vi "SetEmbeddedName.vi"(8 "error in (no error)":errorcluster, 10 "Name":string, 11 "EmbeddedSMO in":refnum<class "EmbeddedSMO.lvclass">) -> (0 "error out":errorcluster, 3 "EmbeddedSMO out":refnum<class "EmbeddedSMO.lvclass">)   [LabVIEW 2016, in "EmbeddedSMO.lvclass"]
uses:
  EmbeddedSMO.lvclass
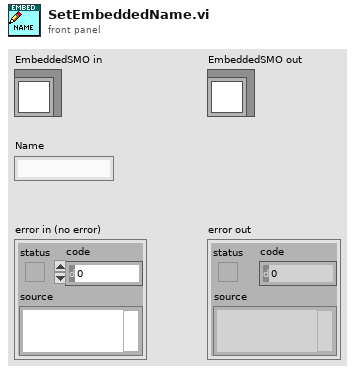
[diagram p1: front panel]
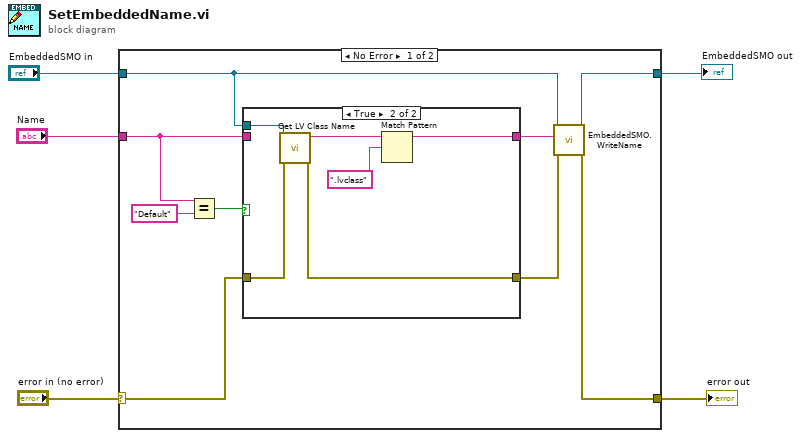
[diagram p0: block diagram]
diagram:
  n1 = case shown="No Error" "error in (no error)" {
    selector: "error in (no error)" -> [w7 w24]
    tunnel: "Name" -> [w10 _]
    tunnel: "EmbeddedSMO in" -> [w8 w23]
    tunnel: [w14 w23] -> w3
    tunnel: [w13 w24] -> w2
    frame No Error {
      n2 = Equal?(x=w10, y="Default") -> (x = y?=w9:bool)
      n3 = case shown="True" w9 {
        tunnel: [w16 w18] -> w11
        tunnel: w10 -> [w16 _]
        tunnel: w8 -> [_ w20]
        tunnel: w7 -> [w15 w22]
        tunnel: [w15 w21] -> w6
        frame False {
        }
        frame True {
          n4 = call <vilib>:"Get LV Class Name.vi"("error in (no error)"=w22, "object"=w20) -> ("error out"=w21:errorcluster, "class name"=w19:string)  [unwired: 8 in]
          n5 = Match Pattern(string=w19, regular expression=".lvclass") -> (before substring=w18:string)  [unwired: 1 in, 3 out]
        }
      }
      n6 = call "EmbeddedSMO.WriteName.vi"("error in (no error)"=w6, "WriteName"=w11, "EmbeddedSMO"=w8) -> ("error out"=w13:errorcluster, "EmbeddedSMO out"=w14:refnum<class "EmbeddedSMO.lvclass">)  [unwired: 7 in]
    }
    frame Error {
    }
  }
  "error out" <- w2
  "EmbeddedSMO out" <- w3
